vi "AcquisitionInterface.vi"() -> ()   [LabVIEW 2025]
uses:
  <vilib>/DAQmx/read.llb/DAQmx Read (Analog 1D Wfm NChan NSamp).vi
  <vilib>/DAQmx/miscellaneous.llb/DAQmx Fill In Error Info.vi
  <vilib>/Waveform/WDTOps.llb/WDT Append Waveforms DBL.vi
panel:
  in  "channel settings":T1={"units"=10348, "input terminal configuration"=10083, "maximum value"=1.5, "minimum value"=-1.5} {"units" items=["Volts"=10348, "From Custom Scale"=10065]; "input terminal configuration" items=["Default"=-1, "RSE"=10083, "NRSE"=10078, "Differential"=10106, "Pseudodifferential"=12529]}
  in  "Max Y value":dbl(slide)=2.5196850393700787 min=0.0 max=10.0 scale=0.0..10.0
  in  "frequency settings":T2={"frequency (Hz)"=1000.0, "number of samples per cycle"=50.0, "number of cycles"=1.0}
  out "file path out":path
  out "error out":errorcluster
  in  "Save to txt":bool
  in  "stop":bool
  out "data":waveform(dbl)(graph)
  in  "error in":errorcluster
  in  "physical channels":tag
  # "La señal se ha guardado en:"
  # "Pulsa este botón para que la señal medida se guarde en un archivo .txt"
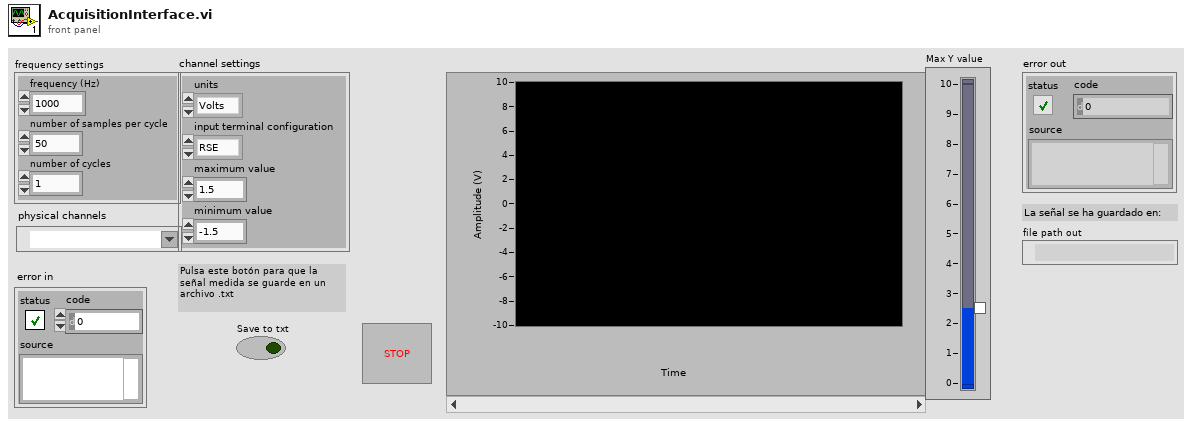
[diagram p1: front panel]
types:
  T1 = cluster{"units":i32, "input terminal configuration":i32, "maximum value":dbl, "minimum value":dbl}
  T2 = cluster{"frequency (Hz)":dbl, "number of samples per cycle":dbl, "number of cycles":dbl}
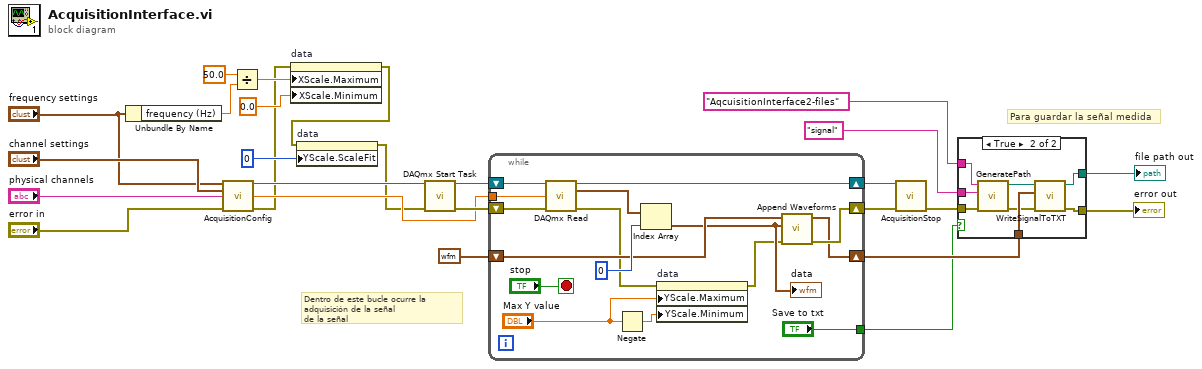
[diagram p0: block diagram]
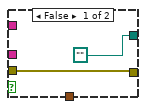
[diagram p2: hidden frame]
diagram:
  # "Para guardar la señal medida"
  # "Dentro de este bucle ocurre la adquisición de la señal\nde la señal"
  n1 = Unbundle By Name("frequency settings") -> ("frequency (Hz)"=w13:dbl)
  n2 = call "AcquisitionConfig.vi"("frequency settings"="frequency settings", "channel settings"="channel settings", "physical channels"="physical channels", "error in"="error in") -> ("task out"=w25:refnum<k21>, "number of samples"=w19:dbl, "error out"=w7:errorcluster)  [unwired: 9 in]
  n3 = Divide(x=50.0, y=w13) -> (x/y=w12:dbl)
  n4 = property on="data" class="WFChart (strict)"(error in=w7, "XScale.Maximum"=w12, "XScale.Minimum"=0.0 ("X Scale.Range:Minimum")) -> (error out=w4:errorcluster)  [unwired: 1 in, 1 out]
  n5 = property on="data" class="WFChart (strict)"(error in=w4, "YScale.ScaleFit"=u8 0 ("Y Scale.Scale Fit")) -> (error out=w6:errorcluster)  [unwired: 1 in, 1 out]
  n6 = call <vilib>:"DAQmx Start Task.vi"("task/channels in"=w25, "error in"=w6) -> ("task out"=w23:refnum<k21>, "error out"=w24:errorcluster)  [unwired: 12 in]
  n7 = while {
    tunnel: w19 -> [w40]
    shift-right: [w34] -> w22
    shift-left: w24 -> [w35]
    shift-right: [w41] -> w21
    shift-left: w23 -> [w42]
    shift-right: [w32] -> w17
    shift-left: waveform(dbl) {"t0"=timestamp(0 s since 1904-01-01), "dt"=1.0, "Y"=[]} ("waveform out") -> [w36]
    tunnel: ["Save to txt"] -> w5
    stop <- "stop" stop-if-true
    n8 = call-poly <vilib>:"DAQmx Read.vi"("task/channels in"=w42, "number of samples per channel"=w40, "error in"=w35) -> ("task out"=w41:refnum<k21>, "data"=w37:waveform(dbl)[], "error out"=w31:errorcluster)  [unwired: 10 in]
    n9 = Negate(x="Max Y value") -> (-x=w30:dbl)
    n10 = Index Array(array=w37, index=0) -> (element=w33:waveform(dbl))
    "data" <- w33
    n11 = property on="data" class="WFChart (strict)"(error in=w31, "YScale.Maximum"="Max Y value", "YScale.Minimum"=w30) -> (error out=w28:errorcluster)  [unwired: 1 in, 1 out]
    n12 = call-poly <vilib>:"Append Waveforms.vi"("error in (no error)"=w28, "waveform B"=w33, "waveform A"=w36) -> ("error out"=w34:errorcluster, "waveform out"=w32:waveform(dbl))  [unwired: 7 in]
  }
  n13 = call "AcquisitionStop.vi"("task/channels in"=w21, "error in"=w22) -> ("error out"=w1:errorcluster)  [unwired: 13 in]
  n14 = case shown="True" w5 {
    tunnel: w17 -> [_ w52]
    tunnel: [w43 w51] -> w16
    tunnel: [path "" w50] -> w15
    tunnel: "AqcuisitionInterface2-files" ("folder  name") -> [_ w49]
    tunnel: "signal" ("file name (no extension)") -> [_ w48]
    tunnel: w1 -> [w43 w47]
    frame False {
    }
    frame True {
      n15 = call "GeneratePath.vi"("error in (no error)"=w47, "file name (no extension)"=w48, "folder  name"=w49) -> ("error out"=w45:errorcluster, "path"=w46:path)  [unwired: 7 in]
      n16 = call "WriteSignalToTXT.vi"("error in"=w45, "waveform"=w52, "file path in"=w46) -> ("error out"=w51:errorcluster, "file path out"=w50:path)  [unwired: 7 in]
    }
  }
  "error out" <- w16
  "file path out" <- w15
